vi "Motion Model - Standalone Main.vi"() -> ()   [LabVIEW 2021]
uses:
  Lab 5/Lab 5 Code/Heading_TDef.ctl
  Main - States_SubVI.ctl
  <vilib>/Platform/TimedLoop/XDataNode/timing_clust.ctl
  <vilib>/Platform/TimedLoop/XDataNode/nitl_modes.ctl
  <vilib>/Platform/TimedLoop/XDataNode/wakeup.ctl
  ProducerConsumer Data Cluster_TDef.ctl
  Measurement Data Cluster_TDef.ctl
  <vilib>/platform/TimedLoop/XDataNode/XDataNode.xnode
  <vilib>/Platform/TimedLoop/XDataNode/XDNodeRunTimeDep.lvlib
  <vilib>/Simulation/Implementation/XNodeFramework/SimXNode/SimX.xnode
  <vilib>/Simulation/Estimation/Implementation/NILVSim Discrete Kalman Filter.llb/SIM Disc KF Pred and Corr with Pred Gain with Checking Direct LV.vi
  <vilib>/addons/Control Design/_Stochastic Systems/Stochastic Systems.llb/Stochastic Systems SubVIs/cd_Stochastic State-Space Model.ctl
  <vilib>/addons/Control Design/_Stochastic Systems/NI_CD_Stochastic Systems.lvlib
panel:
  out "XY Graph 2":T1(graph)
  out "Producer Loop Time (ms)":i32
  out "Consumer Loop Time (ms)":i32
  out "DIP State":T2
  out "Time Elapsed (min)":dbl
  out "North":dbl
  out "East":dbl
  out "Heading String 2":T3
  out "Heading":dbl
  out "Steps":i32
  in  "error in (no error)":errorcluster
  in  "Reset Gyro":bool
  out "Acceleration (g)":T4(graph)
  out "Velocity":T5(graph)
  out "Rotation":T4(graph)
  out "Acceleration (ms^2)":dbl[](array[numeric])
  out "Velocity Cluster Out":cluster{i16, i16, i16}
  out "Rotation Cluster Out":T6
  out "error out":errorcluster
  in  "stop":bool
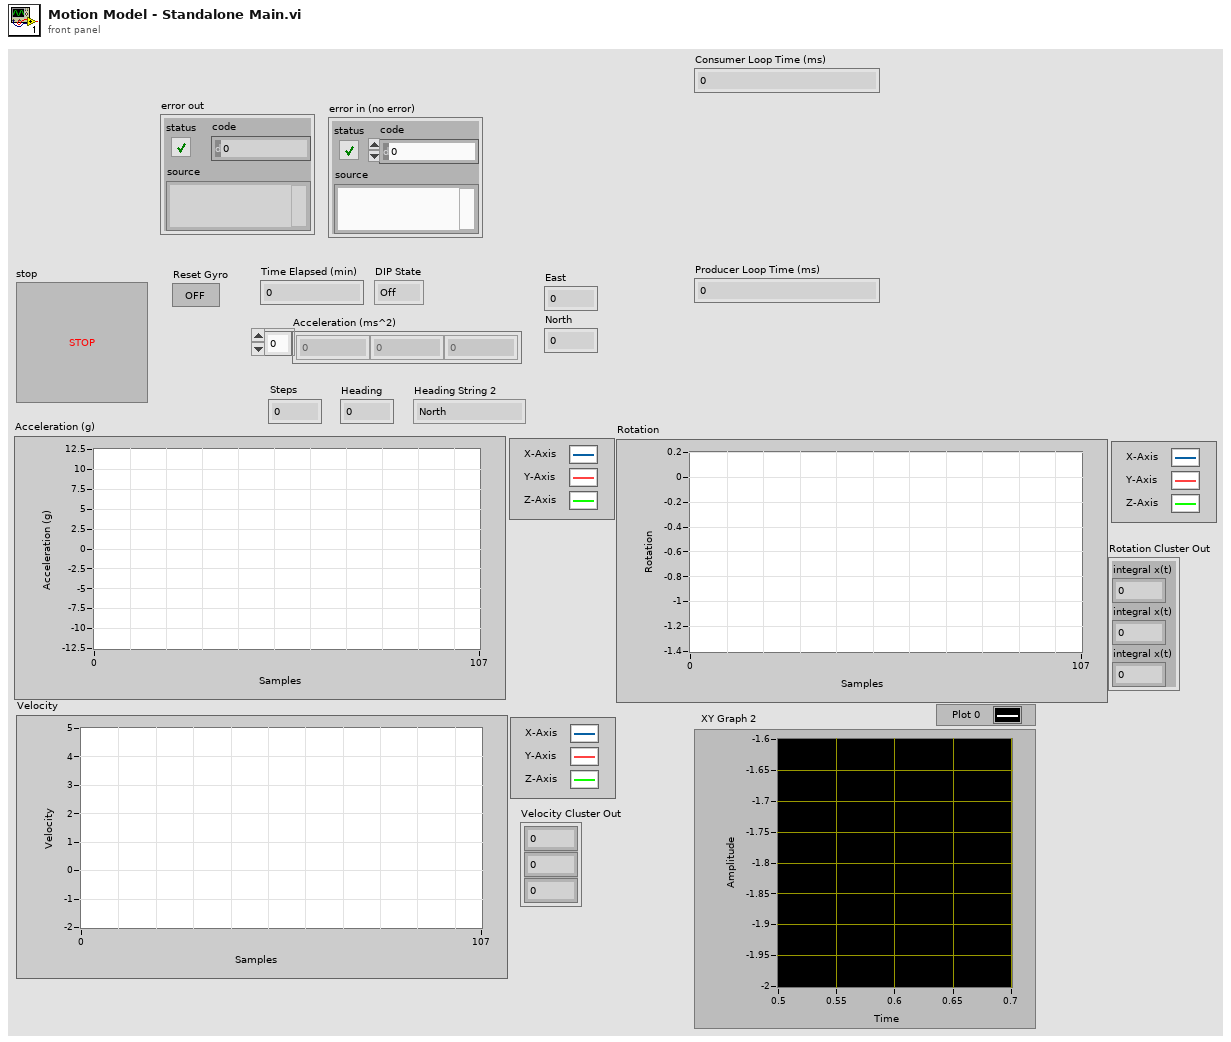
[diagram p1: front panel]
types:
  T1 = cluster{"X Displacement Array ":dbl[], "Y Displacement Array ":dbl[]}
  T2 = typedef "Main - States_SubVI.ctl" = enum16{"Off", "Record", "Upload", "Shutdown", "Error"}
  T3 = typedef "Heading_TDef.ctl" = enum16{"North ", "North East", "East", "Southeast", "South", "Southwest", "West", "Northwest"}
  T4 = cluster{"X-Axis":dbl, "Y-Axis":dbl, "Z-Axis":dbl}
  T5 = cluster{"Velocity":dbl, "Velocity":dbl, "Velocity":dbl}
  T6 = cluster{"integral x(t)":dbl, "integral x(t)":dbl, "integral x(t)":dbl}
  T7 = typedef "Measurement Data Cluster_TDef.ctl" = cluster{"Step Count":i32, "East Displacement":dbl, "North Displacement":dbl, "Longitude":dbl, "Latitude":dbl, "Heart Rate":dbl, "Time Elapsed (min)":dbl}
  T8 = typedef "ProducerConsumer Data Cluster_TDef.ctl" = cluster{"Accelerometer":dbl[], "Gyro":dbl[], "Magnetometer":dbl, "Time":i32, "Pulse":dbl}
  T9 = typedef "XDNodeRunTimeDep.lvlib/timing_clust.ctl" = cluster{"Expected End [f-1]":u64, "Actual End [f-1]":u64, "Finished Late? [f-1]":bool, "Expected End [i-1]":u64, "Actual End [i-1]":u64, "Finished Late? [i-1]":bool, "Expected Start [i]":u64, "Actual Start [i]":u64, "Expected Start [f]":u64, "Actual Start [f]":u64, "Source Name":string, "Structure Name":string, "Period":i64, "Deadline":i64, "Offset":i64, "Start":i64, "Priority":i32, "Timeout":i32, "Mode":T10, "Wakeup Reason":T11, "Error":errorcluster, "Source Type":string, "Secondary Source Type":string, "Global End Time":u64, "Global Start Time":u64, "Frame Duration":u64, "Iteration Duration":u64, "Assigned CPU":i32, "I/O Scan Engine Mode":u32}
  T10 = typedef "XDNodeRunTimeDep.lvlib/nitl_modes.ctl" = enum32{"No Change", "Process missed periods, maintain original phase", "Discard missed periods, maintain original phase", "Process missed periods, ignore original phase", "Discard missed periods, ignore original phase"}
  T11 = typedef "XDNodeRunTimeDep.lvlib/wakeup.ctl" = enum32{"Normal", "Aborted", "Asynchronous wakeup", "Timing source error", "Timed loop error", "Timeout"}
  T12 = typedef "I2C.lvlib/I2C Reference.ctl" = cluster{"myRIO Reference":T13, "I2C Channels Enum":T17, "I2C Configuration":T18}
  T13 = typedef "myRIO Generic Hardware Reference.ctl" = cluster{"myRIO Model":T14, "myRIO Hardware Reference":T15}
  T14 = typedef "Hardware Version Enum.ctl" = enum16{"Unknown", "myRIO-1900", "myRIO-1950", "roboRIO", "NI ELVIS RIO CM", "ELVIS III"}
  T15 = typedef "myRIO v1.0 Reference.ctl" = cluster{"Generic FPGA Reference":T16, "Allow multiple opens":bool}
  T16 = typedef "Generic FPGA Reference.ctl" = refnum<k20>
  T17 = typedef "I2C Channels Enum.ctl" = enum16{"Not Connected", "A/I2C", "B/I2C", "I2C/I2C"}
  T18 = typedef "I2C.lvlib/I2C Configuration.ctl" = cluster{"I2C Transfer Rate":T19}
  T19 = typedef "I2C.lvlib/I2C Transfer Rate.ctl" = enum16{"Standard mode (100 kbps)", "Fast mode (400 kbps)"}
  T20 = typedef "NI_CD_Stochastic Systems.lvlib/cd_Stochastic State-Space Model.ctl" = cluster{"Sampling Time (s)":dbl, "G":dbl[][], "B":dbl[][], "A":dbl[][], "C":dbl[][], "D":dbl[][], "H":dbl[][]}
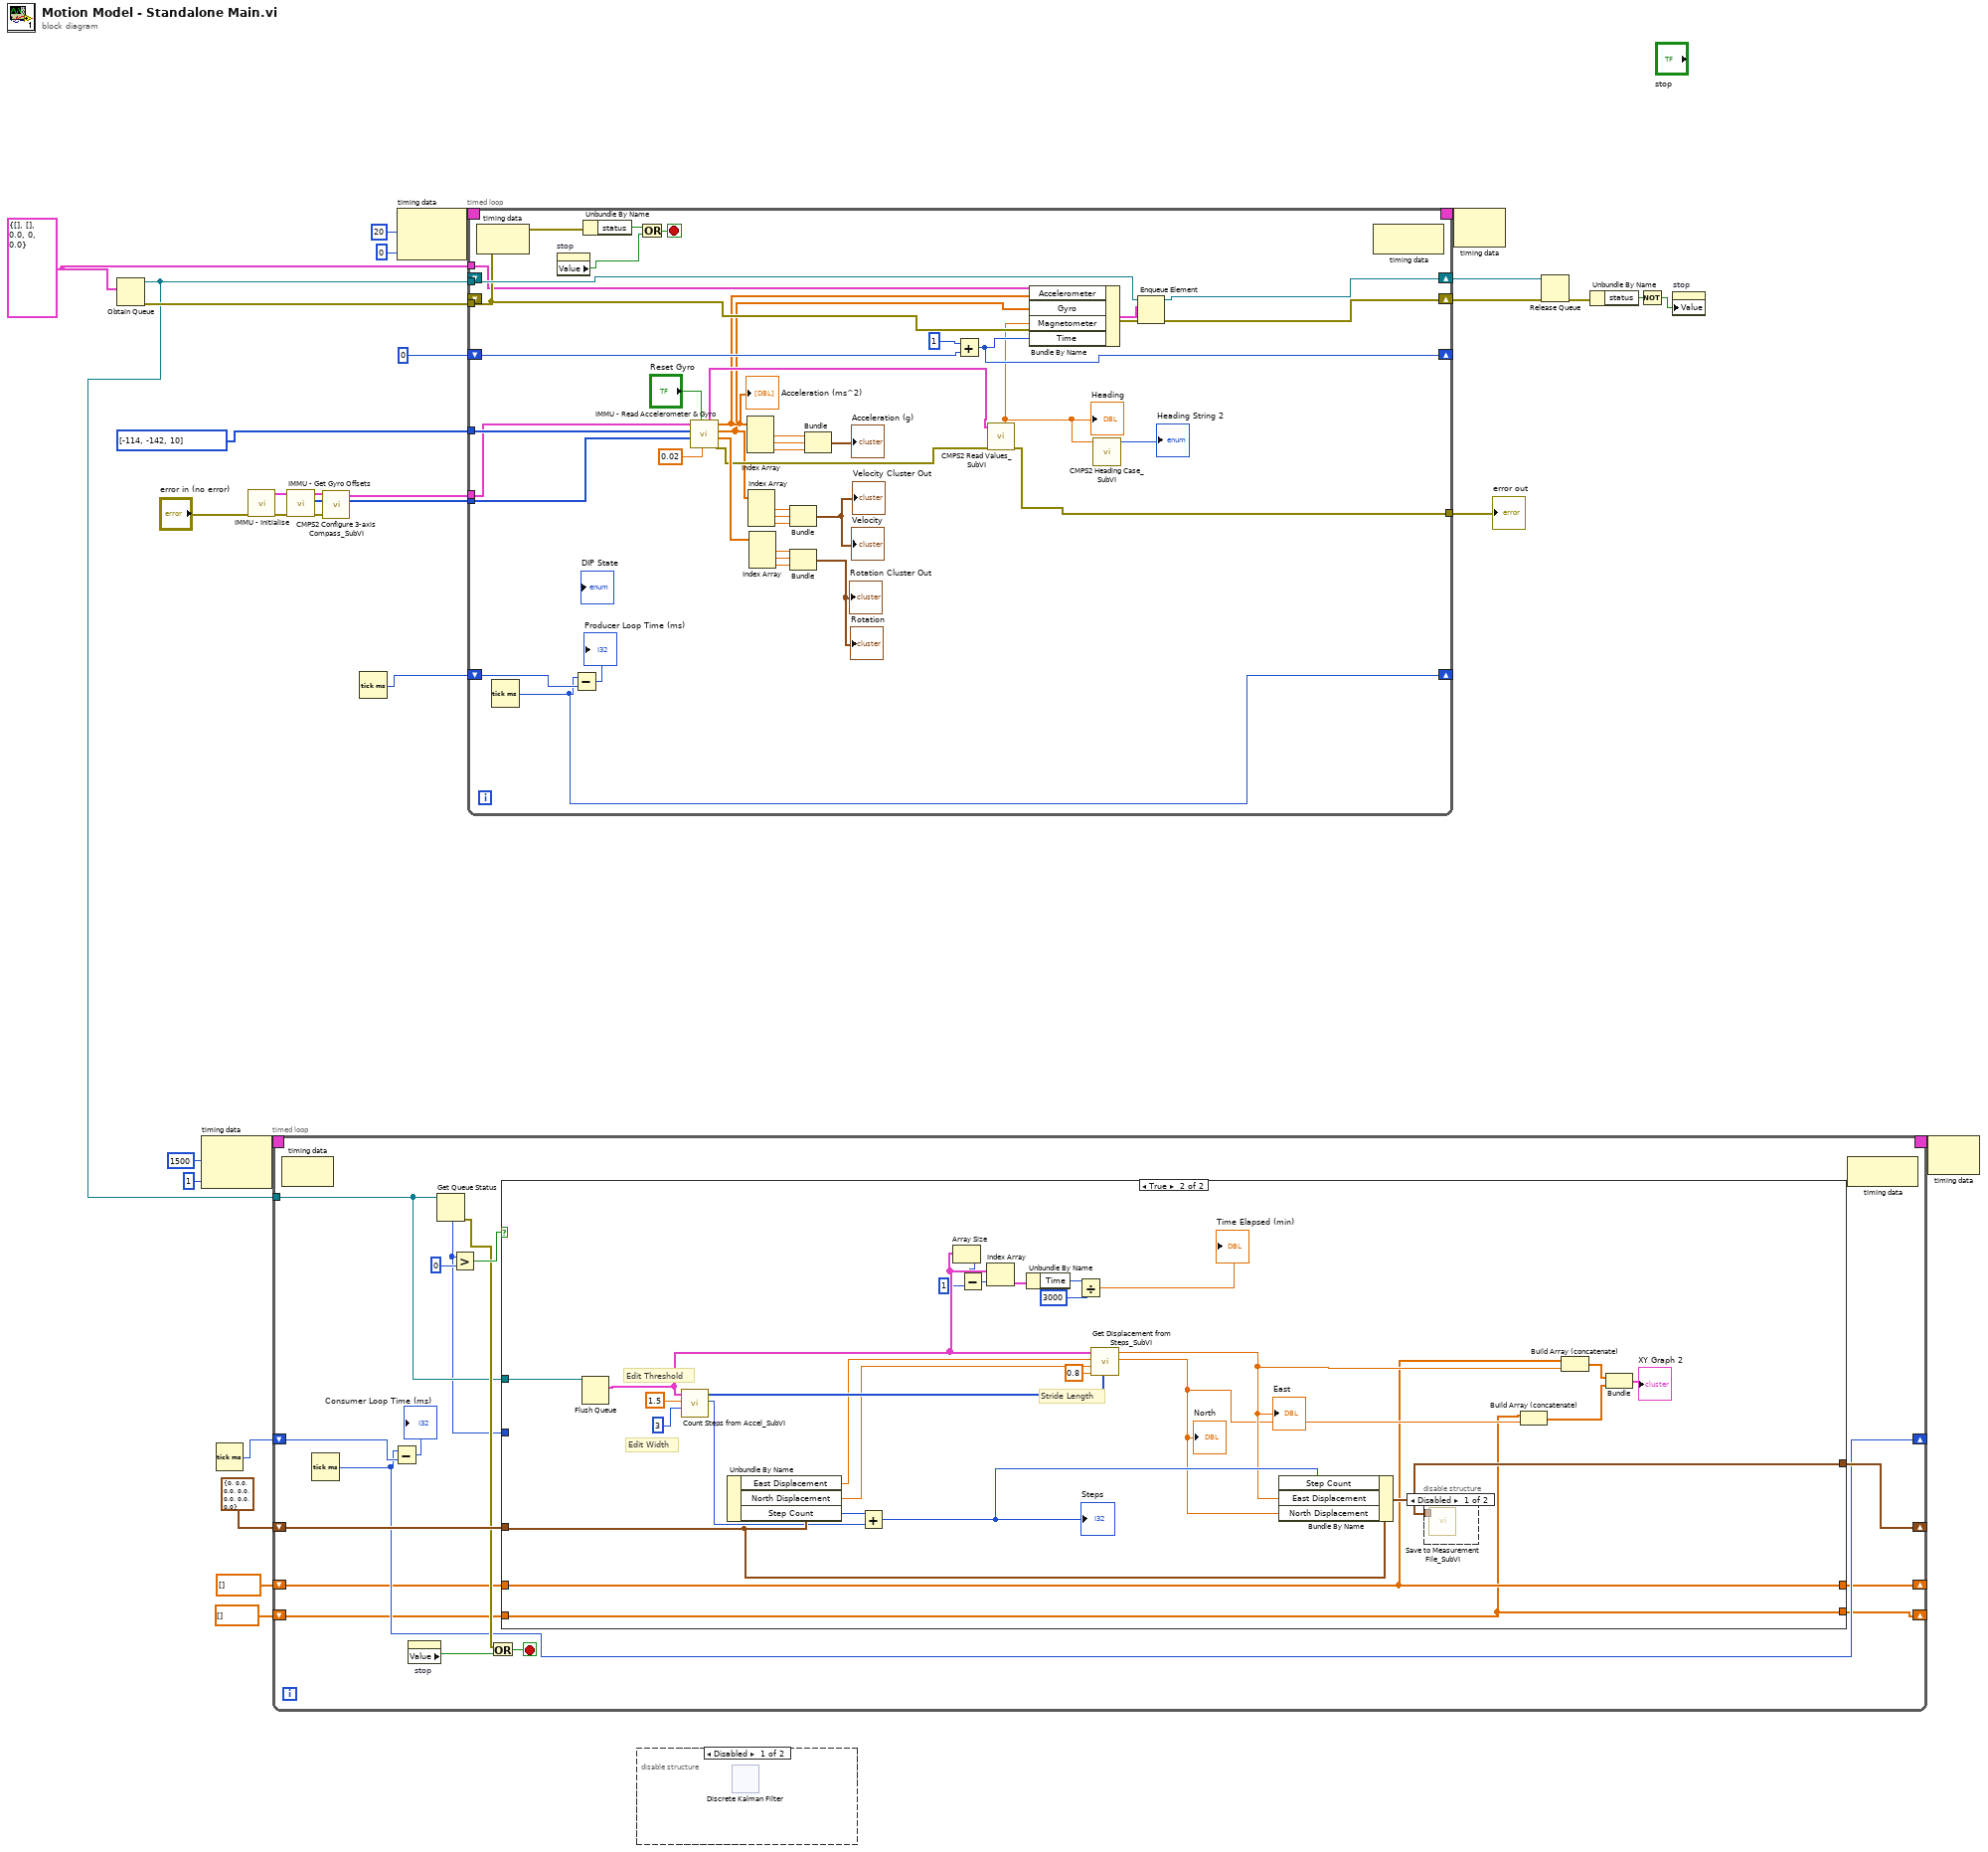
[diagram p0: block diagram]
diagram:
  w8 = T8 {"Accelerometer"=[], "Gyro"=[], "Magnetometer"=0.0, "Time"=0, "Pulse"=0.0}
  n1 = Obtain Queue(element data type=w8) -> (queue out=w23:refnum<queue>, error out=w24:errorcluster)  [unwired: 4 in, 1 out]
  n2 = node-c288(i64 1500 ("Period"), 1 ("Processor")) -> (w29:T9)
  n3 = Tick Count (ms)() -> (millisecond timer value=w4:u32)
  n4 = call "IMMU - Initialise.vi"("error in (no error)"="error in (no error)") -> ("error out"=w18:errorcluster, "I2C Ref Out"=w17:T12)  [unwired: 9 in]
  n5 = timed-loop {
    timing: w29 -> [_]
    timing-out: [_] -> w28
    tunnel: w23 -> [w41]
    shift-right: [w40] -> _
    shift-left: T7 {"Step Count"=0, "East Displacement"=0.0, "North Displacement"=0.0, "Longitude"=0.0, "Latitude"=0.0, "Heart Rate"=0.0, "Time Elapsed (min)"=0.0} -> [w43]
    shift-right: [w36] -> _
    shift-left: w4 -> [w37]
    shift-right: [w33] -> _
    shift-left: dbl[] [] ("threshold") -> [w35]
    shift-right: [w32] -> _
    shift-left: dbl[] [] ("threshold") -> [w34]
    stop <- w46 stop-if-true
    n6 = node-c288() -> ()  [unwired: 1 in, 1 out]
    n7 = Tick Count (ms)() -> (millisecond timer value=w36:u32)
    n8 = Subtract(x=w36, y=w37) -> (x-y=→"Consumer Loop Time (ms)":u32)
    n9 = property on="stop" class="Bool (strict)"() -> ("Value"=w45:bool)  [unwired: 2 in, 2 out]
    n10 = Get Queue Status(queue=w41) -> (error out=w42:errorcluster, # elements in queue=w39:i32)  [unwired: 2 in, 6 out]
    n11 = Greater?(x=w39, y=0) -> (0:w44:bool)
    n12 = Or(x=w42, y=w45) -> (x .or. y?=w46:bool)
    n13 = case shown="True" w44 {
      tunnel: w43 -> [w50 w73]
      tunnel: [w50 w68] -> w40
      tunnel: w41 -> [_ w75]
      tunnel: w39 -> [_ _]
      tunnel: w35 -> [w49 w52]
      tunnel: w34 -> [w48 w51]
      tunnel: [w49 w52] -> w33
      tunnel: [w48 w51] -> w32
      frame False {
      }
      frame True {
        # "Stride Length"
        # "Edit Width"
        # "Edit Threshold"
        n14 = Flush Queue(queue=w75) -> (remaining elements=w63:T8[])  [unwired: 1 in, 2 out]
        n15 = call "Count Steps from Accel_SubVI.vi"("width"=3, "threshold"=1.5, "Queue Elements In"=w63) -> ("Step Count"=w71:i32, "Step Indices"=w72:i32[])  [unwired: 6 in, 1 out]
        n16 = Unbundle By Name(w73) -> ("East Displacement"=w70:dbl, "North Displacement"=w69:dbl, "Step Count"=w74:i32)
        n17 = Add(x=w74, y=w71) -> (x+y=w67:i32)
        "Steps" <- w67
        n18 = Array Size(array=w63) -> (size(s)=w61:i32)
        n19 = Subtract(x=w61, y=1) -> (x-y=w62:i32)
        n20 = Index Array(array=w63, index=w62) -> (element=w66:T8)
        n21 = Unbundle By Name(w66) -> ("Time"=w65:i32)
        n22 = Divide(x=w65, y=3000) -> (x/y=→"Time Elapsed (min)":dbl)
        n23 = call "Get Displacement from Steps_SubVI.vi"("Step Indices"=w72, "Stride Length"=0.8, "North Displacement In"=w69, "East Displacement In"=w70, "Queue Elements In"=w63) -> ("North Displacement Out"=w54:dbl, "East Displacement Out"=w56:dbl)  [unwired: 5 in]
        "East" <- w56
        "North" <- w54
        n24 = Bundle By Name(cluster=w73, "Step Count"=w67, "East Displacement"=w56, "North Displacement"=w54) -> (w68:T7)
        n25 = disable-structure shown="Disabled" {
          disable-tunnel: w68 -> [w78 _]
          frame Disabled {
            n26 = call "Save to Measurement File_SubVI.vi"("Input Cluster Data"=w78) -> ()  [unwired: 10 in, 1 out]
          }
          frame Enabled {
          }
        }
        n27 = Build Array (concatenate)(w51, w54) -> (w53:dbl[])
        n28 = Build Array (concatenate)(w52, w56) -> (w55:dbl[])
        n29 = Bundle(w55, w53) -> (→"XY Graph 2":cluster{dbl[], dbl[]})  [unwired: 1 in]
      }
    }
    n30 = node-c288() -> ()  [unwired: 1 in, 1 out]
  }
  n31 = call "IMMU - Get Gyro Offsets.vi"("error in (no error)"=w18, "I2C Ref In"=w17) -> ("error out"=w10:errorcluster, "Output Offset Array (int)"=w15:i16[], "I2C Ref Out"=w11:T12)  [unwired: 7 in]
  n32 = call "CMPS2 Configure 3-axis Compass_SubVI.vi"("error in (no error)"=w10, "I2C Ref In"=w11) -> ("I2C Ref Out"=w9:T12)  [unwired: 8 in, 1 out]
  n33 = Tick Count (ms)() -> (millisecond timer value=w3:u32)
  n34 = node-c288(i64 20 ("Period"), 0 ("Processor")) -> (w31:T9)
  n35 = timed-loop {
    timing: w31 -> [_]
    timing-out: [_] -> w30
    tunnel: w23 -> [w114]
    tunnel: w24 -> [w113]
    shift-right: [w115] -> w22
    shift-left: _ -> [_]
    shift-right: [w112] -> w21
    shift-left: _ -> [_]
    tunnel: i16[] [-114, -142, 10] ("Accel Offset Array In") -> [w117]
    tunnel: w15 -> [w116]
    tunnel: w9 -> [w111]
    tunnel: w8 -> [w110]
    shift-right: [w108] -> _
    shift-left: 0 -> [w109]
    tunnel: [w81] -> w5
    shift-right: [w105] -> _
    shift-left: w3 -> [w106]
    stop <- w120 stop-if-true
    n36 = node-c288() -> ()  [unwired: 1 in, 1 out]
    n37 = Tick Count (ms)() -> (millisecond timer value=w105:u32)
    n38 = property on="stop" class="Bool (strict)"() -> ("Value"=w118:bool)  [unwired: 2 in, 2 out]
    n39 = Subtract(x=w105, y=w106) -> (x-y=→"Producer Loop Time (ms)":u32)
    n40 = Unbundle By Name(w113) -> ("status"=w119:bool)
    n41 = Or(x=w119, y=w118) -> (x .or. y?=w120:bool)
    n42 = call "IMMU - Read Accelerometer & Gyro.vi"("dt"=0.02, "Reset Gyro"="Reset Gyro", "Gyro Offset Array In"=w116, "Accel Offset Array In"=w117, "I2C Ref In"=w111) -> ("error out"=w90:errorcluster, "Gyro Rotation Out (degrees)"=w100:dbl[], "Gyro Rotational Velocity Out (deg/s)"=w87:dbl[], "Output Acceleration Array (ms^2)"=w88:dbl[], "I2C Ref Out"=w92:T12)  [unwired: 2 in]
    "Acceleration (ms^2)" <- w88
    n43 = Index Array(array=w88) -> (element #1=w99:dbl, element #2=w98:dbl, element #3=w97:dbl)  [unwired: 3 in]
    n44 = Index Array(array=w87) -> (element #1=w96:dbl, element #2=w95:dbl, element #3=w94:dbl)  [unwired: 3 in]
    n45 = Index Array(array=w100) -> (element #1=w104:dbl, element #2=w103:dbl, element #3=w102:dbl)  [unwired: 3 in]
    n46 = Bundle(w96, w95, w94) -> (→"Velocity Cluster Out" →"Velocity":cluster{dbl, dbl, dbl})  [unwired: 1 in]
    n47 = Bundle("integral x(t)"=w104, "integral x(t)"=w103, "integral x(t)"=w102) -> (→"Rotation Cluster Out" →"Rotation":T6)  [unwired: 1 in]
    n48 = Bundle(w99, w98, w97) -> (→"Acceleration (g)":cluster{dbl, dbl, dbl})  [unwired: 1 in]
    n49 = Add(x=1, y=w109) -> (x+y=w108:i32)
    n50 = call "CMPS2 Read Values_SubVI.vi"("error in (no error)"=w90, "I2C Ref In"=w92) -> ("error out"=w81:errorcluster, "Heading"=w86:dbl)  [unwired: 4 in, 4 out]
    "Heading" <- w86
    n51 = Bundle By Name(cluster=w110, "Accelerometer"=w88, "Gyro"=w87, "Magnetometer"=w86, "Time"=w108) -> (w89:T8)
    n52 = call "CMPS2 Heading Case_SubVI.vi"("Numeric"=w86) -> ("Heading String 2"=→"Heading String 2":T3)  [unwired: 10 in]
    n53 = Enqueue Element(queue=w114, element=w89, error in (no error)=w113) -> (queue out=w112:refnum<queue>, error out=w115:errorcluster)  [unwired: 1 in, 1 out]
    n54 = node-c288() -> ()  [unwired: 1 in, 1 out]
  }
  "error out" <- w5
  n55 = disable-structure shown="Disabled" {
    frame Disabled {
      n56 = xnode "Discrete Kalman Filter"() -> ()  [unwired: 4 in, 8 out]
    }
    frame Enabled {
    }
  }
  n57 = node-c288(w30) -> ()  [unwired: 1 out]
  n58 = Release Queue(queue=w21, error in (no error)=w22) -> (error out=w14:errorcluster)  [unwired: 1 in, 2 out]
  n59 = Unbundle By Name(w14) -> ("status"=w13:bool)
  n60 = Not(x=w13) -> (.not. x?=w12:bool)
  n61 = property on="stop" class="Bool (strict)"("Value"=w12) -> ()  [unwired: 2 in, 2 out]
  n62 = node-c288(w28) -> ()  [unwired: 1 out]
